vi "R5TestSomething.vi"() -> ()   [LabVIEW 2016]
panel:
  out "AI31":dbl
  out "AI30":dbl
  out "AI29":dbl
  out "AI28":dbl
  out "AI27":dbl
  out "AI26":dbl
  out "AI25":dbl
  out "AI24":dbl
  out "AI23":dbl
  out "AI22":dbl
  out "AI21":dbl
  out "AI20":dbl
  out "AI19":dbl
  out "AI18":dbl
  out "AI17":dbl
  out "AI16":dbl
  out "AI15":dbl
  out "AI14":dbl
  out "AI13":dbl
  out "AI12":dbl
  out "AI11":dbl
  out "AI10":dbl
  out "AI9":dbl
  out "AI8":dbl
  out "AI7":dbl
  out "AI6":dbl
  out "AI5":dbl
  out "AI4":dbl
  out "AI3":dbl
  out "AI2":dbl
  out "AI1":dbl
  out "AI0":dbl
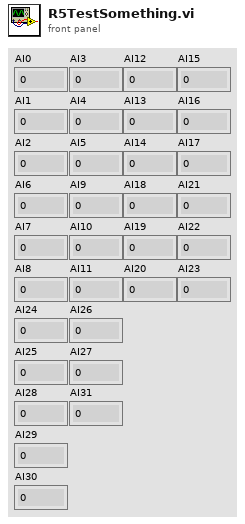
[diagram p1: front panel]
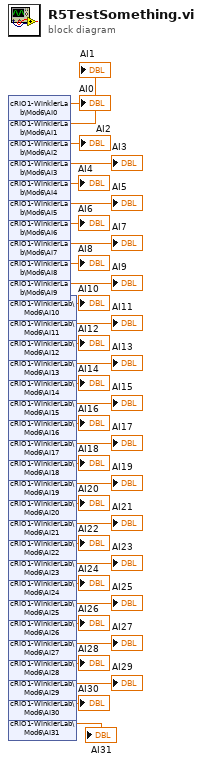
[diagram p0: block diagram]
diagram:
  n1 = shared-variable "cRIO1-WinklerLab\\Mod6\\AI0"() -> (→"AI0":dbl)  [unwired: 1 in, 1 out]
  n2 = shared-variable "cRIO1-WinklerLab\\Mod6\\AI1"() -> (→"AI1":dbl)  [unwired: 1 in, 1 out]
  n3 = shared-variable "cRIO1-WinklerLab\\Mod6\\AI2"() -> (→"AI2":dbl)  [unwired: 1 in, 1 out]
  n4 = shared-variable "cRIO1-WinklerLab\\Mod6\\AI3"() -> (→"AI3":dbl)  [unwired: 1 in, 1 out]
  n5 = shared-variable "cRIO1-WinklerLab\\Mod6\\AI4"() -> (→"AI4":dbl)  [unwired: 1 in, 1 out]
  n6 = shared-variable "cRIO1-WinklerLab\\Mod6\\AI5"() -> (→"AI5":dbl)  [unwired: 1 in, 1 out]
  n7 = shared-variable "cRIO1-WinklerLab\\Mod6\\AI6"() -> (→"AI6":dbl)  [unwired: 1 in, 1 out]
  n8 = shared-variable "cRIO1-WinklerLab\\Mod6\\AI7"() -> (→"AI7":dbl)  [unwired: 1 in, 1 out]
  n9 = shared-variable "cRIO1-WinklerLab\\Mod6\\AI8"() -> (→"AI8":dbl)  [unwired: 1 in, 1 out]
  n10 = shared-variable "cRIO1-WinklerLab\\Mod6\\AI9"() -> (→"AI9":dbl)  [unwired: 1 in, 1 out]
  n11 = shared-variable "cRIO1-WinklerLab\\Mod6\\AI10"() -> (→"AI10":dbl)  [unwired: 1 in, 1 out]
  n12 = shared-variable "cRIO1-WinklerLab\\Mod6\\AI11"() -> (→"AI11":dbl)  [unwired: 1 in, 1 out]
  n13 = shared-variable "cRIO1-WinklerLab\\Mod6\\AI12"() -> (→"AI12":dbl)  [unwired: 1 in, 1 out]
  n14 = shared-variable "cRIO1-WinklerLab\\Mod6\\AI13"() -> (→"AI13":dbl)  [unwired: 1 in, 1 out]
  n15 = shared-variable "cRIO1-WinklerLab\\Mod6\\AI14"() -> (→"AI14":dbl)  [unwired: 1 in, 1 out]
  n16 = shared-variable "cRIO1-WinklerLab\\Mod6\\AI15"() -> (→"AI15":dbl)  [unwired: 1 in, 1 out]
  n17 = shared-variable "cRIO1-WinklerLab\\Mod6\\AI16"() -> (→"AI16":dbl)  [unwired: 1 in, 1 out]
  n18 = shared-variable "cRIO1-WinklerLab\\Mod6\\AI17"() -> (→"AI17":dbl)  [unwired: 1 in, 1 out]
  n19 = shared-variable "cRIO1-WinklerLab\\Mod6\\AI18"() -> (→"AI18":dbl)  [unwired: 1 in, 1 out]
  n20 = shared-variable "cRIO1-WinklerLab\\Mod6\\AI19"() -> (→"AI19":dbl)  [unwired: 1 in, 1 out]
  n21 = shared-variable "cRIO1-WinklerLab\\Mod6\\AI20"() -> (→"AI20":dbl)  [unwired: 1 in, 1 out]
  n22 = shared-variable "cRIO1-WinklerLab\\Mod6\\AI21"() -> (→"AI21":dbl)  [unwired: 1 in, 1 out]
  n23 = shared-variable "cRIO1-WinklerLab\\Mod6\\AI22"() -> (→"AI22":dbl)  [unwired: 1 in, 1 out]
  n24 = shared-variable "cRIO1-WinklerLab\\Mod6\\AI23"() -> (→"AI23":dbl)  [unwired: 1 in, 1 out]
  n25 = shared-variable "cRIO1-WinklerLab\\Mod6\\AI24"() -> (→"AI24":dbl)  [unwired: 1 in, 1 out]
  n26 = shared-variable "cRIO1-WinklerLab\\Mod6\\AI25"() -> (→"AI25":dbl)  [unwired: 1 in, 1 out]
  n27 = shared-variable "cRIO1-WinklerLab\\Mod6\\AI26"() -> (→"AI26":dbl)  [unwired: 1 in, 1 out]
  n28 = shared-variable "cRIO1-WinklerLab\\Mod6\\AI27"() -> (→"AI27":dbl)  [unwired: 1 in, 1 out]
  n29 = shared-variable "cRIO1-WinklerLab\\Mod6\\AI28"() -> (→"AI28":dbl)  [unwired: 1 in, 1 out]
  n30 = shared-variable "cRIO1-WinklerLab\\Mod6\\AI29"() -> (→"AI29":dbl)  [unwired: 1 in, 1 out]
  n31 = shared-variable "cRIO1-WinklerLab\\Mod6\\AI30"() -> (→"AI30":dbl)  [unwired: 1 in, 1 out]
  n32 = shared-variable "cRIO1-WinklerLab\\Mod6\\AI31"() -> (→"AI31":dbl)  [unwired: 1 in, 1 out]
